vi "Reset Cursors Center.vi"(8 "Error In":errorcluster, 11 "Waveform Graph":refnum<vi>) -> (0 "error out":errorcluster)   [LabVIEW 2017]
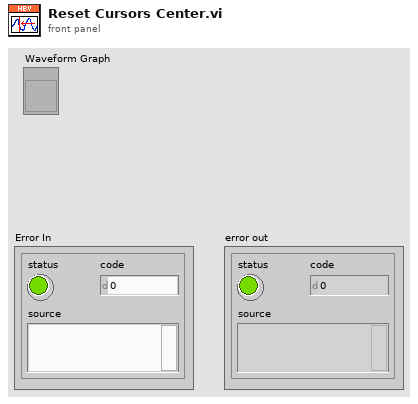
[diagram p1: front panel]
types:
  T1 = typedef "LVCursorListTypeDef.ctl" = cluster{"Name":string, "Color":u32, "Style":u8, "Point Style":u8, "Name Visible":bool, "Allow Drag":bool, "Cursor Mode":u32, "Plot":i32, "Index":i32, "Position":cluster{"X":dbl, "Y":dbl}, "X Scale":u32, "Y Scale":u32, "Watch Plots":i32[], "Watch All Plots":bool, "Plot Area":i32, "Label Offset":cluster{"X":dbl, "Y":dbl}}[]
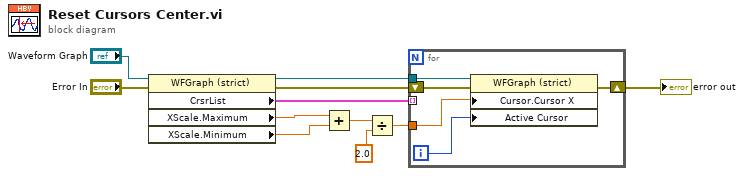
[diagram p0: block diagram]
diagram:
  n1 = property class="WFGraph (strict)"(reference="Waveform Graph", error in="Error In") -> (reference out=w6:refnum<vi>, error out=w8:errorcluster, "CrsrList"=w7:T1, "XScale.Maximum"=w5:dbl, "XScale.Minimum"=w4:dbl)
  n2 = Add(x=w5, y=w4) -> (x+y=w3:dbl)
  n3 = Divide(x=w3, y=2.0) -> (x/y=w1:dbl)
  n4 = for {
    tunnel: w7 -> [_] mode=indexing
    tunnel: w6 -> [w16]
    shift-right: [w14] -> w11
    shift-left: w8 -> [w13]
    tunnel: w1 -> [w12]
    i -> [w15]
    n5 = property class="WFGraph (strict)"(reference=w16, error in=w13, "Cursor.Cursor X"=w12, "Active Cursor"=w15) -> (error out=w14:errorcluster)  [unwired: 1 out]
  }
  "error out" <- w11
